vi "NMRvmefull3.vi"() -> ()   [LabVIEW 2013]
uses:
  <vilib>/Utility/file.llb/Read From Spreadsheet File (DBL).vi
  <vilib>/Analysis/NI_AALBase.lvlib
panel:
  in  "Real/quad Q curve":bool=TRUE
  out "Temperature":dbl(graph)=22.5
  out "+3V supply":dbl=3.026 format="%_4g"
  out "Temp (C)":dbl=22.5 format="%_4g"
  in  "RemovePed":bool=TRUE
  in  "IF / LOG Det":bool
  in  "Q curve file":string="realback213.txt"
  out "File name 2":string="C:\\users\\plm\\Desktop\\rssmt\\realback213.txt"
  in  "AutoBaseline":bool=TRUE
  out "RF OK":bool=TRUE
  out "Peak area (V-MHz)":sgl=0.008512556 format="%.5f"
  in  "Gauss Fit":bool=TRUE
  out "NMR Graph + Fit":cluster{cluster{dbl, "Numeric":dbl}[]}[](graph)=[{[{224.37, "Numeric"=-0.000659019047619289}, {224.372, "Numeric"=-0.001187546666660903}, {224.374, "Numeric"=-0.003239274285720313}, {224.376, "Numeric"=-0.004214201904762039}, {224.37800000000001, "Numeric"=-0.002912329523803976}, {224.38, "Numeric"=-0.007933657142862722}, {224.382, "Numeric"=-0.005878184761904778}, {224.38400000000001, "Numeric"=-0.00914591238094707}, {224.386, "Numeric"=-0.00463684000000517}, {224.388, "Numeric"=-0.0009509676190475541}, {224.39000000000001, "Numeric"=-0.004488295238090173}, {224.392, "Numeric"=-0.004948822857147612}, {224.394, "Numeric"=-0.0035325504761903404}, {224.39600000000002, "Numeric"=-0.0007394780952332926}, {224.398, "Numeric"=0.0009303942857099255}, {224.4, "Numeric"=0.004277066666666864}, {224.40200000000002, "Numeric"=0.0017005390476235753}, {224.404, "Numeric"=0.0039008114285674464}, {224.406, "Numeric"=0.003777883809524034}, {224.40800000000002, "Numeric"=0.004031756190480424}, {224.41, "Numeric"=0.0019624285714249347}, {224.412, "Numeric"=0.00796990095238121}, {224.41400000000002, "Numeric"=5.417333333726862e-05}, {224.416, "Numeric"=0.0012152457142824398}, {224.418, "Numeric"=-0.0023468819047616283}, {224.42000000000002, "Numeric"=-0.00023220952380592283}, {224.422, "Numeric"=0.003659262857139909}, {224.424, "Numeric"=0.0047275352380955005}, {224.426, "Numeric"=0.008272607619049287}, {224.428, "Numeric"=0.008894479999997358}, {224.43, "Numeric"=0.011693152380952624}, {224.432, "Numeric"=0.01246862476190608}, {224.434, "Numeric"=0.0106208971428548}, {224.436, "Numeric"=0.012149969523809723}, {224.438, "Numeric"=0.01675584190476286}, {224.44, "Numeric"=0.02263851428571223}, {224.442, "Numeric"=0.026497986666666827}, {224.444, "Numeric"=0.03243425904761961}, {224.446, "Numeric"=0.04374733142856964}, {224.448, "Numeric"=0.0529372038095239}, {224.45, "Numeric"=0.06540387619047636}, {224.452, "Numeric"=0.07984734857142704}, {224.454, "Numeric"=0.09986762095238097}, {224.456, "Numeric"=0.11866469333333307}, {224.458, "Numeric"=0.15183856571428445}, {224.46, "Numeric"=0.19398923809523802}, {224.462, "Numeric"=0.24311671047618982}, {224.464, "Numeric"=0.30252098285714174}, {224.466, "Numeric"=0.347502055238095}, {224.468, "Numeric"=0.3777599276190465}, {224.47, "Numeric"=0.3782945999999991}, {224.472, "Numeric"=0.35440607238095206}, {224.474, "Numeric"=0.29719434476190315}, {224.476, "Numeric"=0.24975941714285646}, {224.478, "Numeric"=0.19870128952380905}, {224.48, "Numeric"=0.16101996190475984}, {224.482, "Numeric"=0.13171543428571375}, {224.484, "Numeric"=0.10748770666666604}, {224.486, "Numeric"=0.08753677904761648}, {224.488, "Numeric"=0.0769626514285711}, {224.49, "Numeric"=0.06146532380952299}, {224.492, "Numeric"=0.05464479619047311}, {224.494, "Numeric"=0.04340106857142838}, {224.496, "Numeric"=0.041234140952379955}, {224.498, "Numeric"=0.034844013333334194}, {224.5, "Numeric"=0.02723068571428565}, {224.502, "Numeric"=0.02559415809523689}, {224.504, "Numeric"=0.015134430476191776}, {224.506, "Numeric"=0.017151502857142897}, {224.508, "Numeric"=0.013645375238093822}, {224.51, "Numeric"=0.008016047619049357}, {224.512, "Numeric"=0.015663520000000142}, {224.514, "Numeric"=0.01228779238095072}, {224.516, "Numeric"=0.005288864761906909}, {224.518, "Numeric"=0.010166737142857376}, {224.51999999999998, "Numeric"=0.007321409523806038}, {224.522, "Numeric"=0.008652881904764452}, {224.524, "Numeric"=0.003961154285714588}, {224.52599999999998, "Numeric"=0.004446226666662913}, {224.528, "Numeric"=0.002708099047621988}, {224.53, "Numeric"=-0.0015532285714282253}, {224.53199999999998, "Numeric"=0.0016622438095197614}, {224.534, "Numeric"=-0.00014548380952048717}, {224.536, "Numeric"=-0.002276411428571029}, {224.53799999999998, "Numeric"=6.946095237661282e-05}, {224.54, "Numeric"=0.00029213333333700424}, {224.542, "Numeric"=0.001291605714286121}, {224.54399999999998, "Numeric"=0.003967878095233438}, {224.546, "Numeric"=-0.0030790495238055193}, {224.548, "Numeric"=-0.0037491771428567293}, {224.54999999999998, "Numeric"=-0.0031425047619097436}, {224.552, "Numeric"=-0.005059032380948048}, {224.554, "Numeric"=-0.006498759999999599}, {224.55599999999998, "Numeric"=-0.0052616876190529505}, {224.558, "Numeric"=-0.005247815238090598}, {224.56, "Numeric"=-0.008557142857142475}, {224.56199999999998, "Numeric"=0.0013103295238038309}, {224.564, "Numeric"=-0.0059453980952331505}, {224.566, "Numeric"=-0.005024325714285373}, {224.56799999999998, "Numeric"=-0.006226453333339399}, {224.57, "Numeric"=-0.01565178095237573}]}, {[{224.37, "Numeric"=1.2216920919387119e-26}, {224.372, "Numeric"=1.2707531124356022e-25}, {224.374, "Numeric"=1.2602215540394123e-24}, {224.376, "Numeric"=1.1915682596026088e-23}, {224.37800000000001, "Numeric"=1.074180467048424e-22}, {224.38, "Numeric"=9.232554443628677e-22}, {224.382, "Numeric"=7.565764268347757e-21}, {224.38400000000001, "Numeric"=5.911123533707065e-20}, {224.386, "Numeric"=4.403252266347702e-19}, {224.388, "Numeric"=3.1272557579616753e-18}, {224.39000000000001, "Numeric"=2.1175785840334696e-17}, {224.392, "Numeric"=1.3671053194326456e-16}, {224.394, "Numeric"=8.414933959385655e-16}, {224.39600000000002, "Numeric"=4.9383941847663025e-15}, {224.398, "Numeric"=2.7631667539992904e-14}, {224.4, "Numeric"=1.474058566437982e-13}, {224.40200000000002, "Numeric"=7.497365525223633e-13}, {224.404, "Numeric"=3.635707470038474e-12}, {224.406, "Numeric"=1.6809526567726662e-11}, {224.40800000000002, "Numeric"=7.409831514948406e-11}, {224.41, "Numeric"=3.114207067787316e-10}, {224.412, "Numeric"=1.2478803346260637e-09}, {224.41400000000002, "Numeric"=4.7674340851587536e-09}, {224.416, "Numeric"=1.7365318588608352e-08}, {224.418, "Numeric"=6.030691537295004e-08}, {224.42000000000002, "Numeric"=1.99681475508499e-07}, {224.422, "Numeric"=6.303688449783224e-07}, {224.424, "Numeric"=1.897308734090218e-06}, {224.426, "Numeric"=5.4446199856763875e-06}, {224.428, "Numeric"=1.489647258961794e-05}, {224.43, "Numeric"=3.885846244500032e-05}, {224.432, "Numeric"=9.664381932133422e-05}, {224.434, "Numeric"=0.0002291653005566002}, {224.436, "Numeric"=0.000518095636666997}, {224.438, "Numeric"=0.001116753474559677}, {224.44, "Numeric"=0.0022950438712561385}, {224.442, "Numeric"=0.004496876629042055}, {224.444, "Numeric"=0.008400734433419424}, {224.446, "Numeric"=0.014962695593284949}, {224.448, "Numeric"=0.025409067505081276}, {224.45, "Numeric"=0.04113901748058781}, {224.452, "Numeric"=0.06350463222880787}, {224.454, "Numeric"=0.09346374892359874}, {224.456, "Numeric"=0.1311496966920382}, {224.458, "Numeric"=0.1754598225609385}, {224.46, "Numeric"=0.2238073695319673}, {224.462, "Numeric"=0.2721807344877579}, {224.464, "Numeric"=0.31559250621481655}, {224.466, "Numeric"=0.3488849894624623}, {224.468, "Numeric"=0.3677258738997204}, {224.47, "Numeric"=0.36953229107129204}, {224.472, "Numeric"=0.354051877915298}, {224.474, "Numeric"=0.3234206247194692}, {224.476, "Numeric"=0.28167922867646705}, {224.478, "Numeric"=0.23389893037116466}, {224.48, "Numeric"=0.18517738653314392}, {224.482, "Numeric"=0.13977643736304876}, {224.484, "Numeric"=0.10059265830727328}, {224.486, "Numeric"=0.06902158134856975}, {224.488, "Numeric"=0.04515333441124985}, {224.49, "Numeric"=0.028163138467571368}, {224.492, "Numeric"=0.016747831227365746}, {224.494, "Numeric"=0.009495599803450215}, {224.496, "Numeric"=0.005133014978954904}, {224.498, "Numeric"=0.0026455072873873718}, {224.5, "Numeric"=0.0012999651045567388}, {224.502, "Numeric"=0.0006090328646084895}, {224.504, "Numeric"=0.0002720420660815896}, {224.506, "Numeric"=0.00011585577912496795}, {224.508, "Numeric"=4.704198526856143e-05}, {224.51, "Numeric"=1.8211255302093487e-05}, {224.512, "Numeric"=6.721720126132654e-06}, {224.514, "Numeric"=2.3654145853830547e-06}, {224.516, "Numeric"=7.936342772979279e-07}, {224.518, "Numeric"=2.5387495830503464e-07}, {224.51999999999998, "Numeric"=7.742935028573666e-08}, {224.522, "Numeric"=2.251529631140118e-08}, {224.524, "Numeric"=6.2421761553258384e-09}, {224.52599999999998, "Numeric"=1.6499875819670289e-09}, {224.528, "Numeric"=4.1582599244703297e-10}, {224.53, "Numeric"=9.99145856172782e-11}, {224.53199999999998, "Numeric"=2.2889296881634745e-11}, {224.534, "Numeric"=4.999450980324916e-12}, {224.536, "Numeric"=1.0411144604004796e-12}, {224.53799999999998, "Numeric"=2.0670974178453588e-13}, {224.54, "Numeric"=3.9129987765540336e-14}, {224.542, "Numeric"=7.062277550488454e-15}, {224.54399999999998, "Numeric"=1.215251463338106e-15}, {224.546, "Numeric"=1.9937643473100612e-16}, {224.548, "Numeric"=3.1186583504921976e-17}, {224.54999999999998, "Numeric"=4.6510186053397055e-18}, {224.552, "Numeric"=6.613245651569734e-19}, {224.554, "Numeric"=8.965355910234511e-20}, {224.55599999999998, "Numeric"=1.1587952779623013e-20}, {224.558, "Numeric"=1.4280131290425803e-21}, {224.56, "Numeric"=1.6778146633486307e-22}, {224.56199999999998, "Numeric"=1.8794988861895673e-23}, {224.564, "Numeric"=2.0073655264081265e-24}, {224.566, "Numeric"=2.0440765317757311e-25}, {224.56799999999998, "Numeric"=1.984513896750819e-26}, {224.57, "Numeric"=1.8369504363521433e-27}]}]
  in  "Amp of Q curve":dbl=2.899999999999994 min=0.0 max=3.0 step=0.01 format="%_3f"
  in  "Subtract Q curve":bool=TRUE
  in  "Adjust Tune":bool
  out "Ped Offset":dbl(graph)=0.06850250000000084
  out "Pedestal Difference":dbl(graph)=-0.007803066666666664
  out "# Good Spectra":i32=29509
  in  "Quality cuts":bool=TRUE
  out "Pedestal OK":bool=TRUE
  out "Sweep #":i32=45
  out "1st Sweep":bool
  out "ADC volts OK":bool=TRUE
  out "Peak Height Distribution":cluster{"Y":dbl[], "Y":dbl[]}[](graph)=[{"Y"=[0.34871442808966735, 0.3488976491432983, 0.3490808701969293, 0.3492640912505603, 0.34944731230419124, 0.34963053335782224, 0.34981375441145324, 0.3499969754650842, 0.3501801965187152, 0.3503634175723462, 0.3505466386259771, 0.3507298596796081, 0.3509130807332391, 0.35109630178687007, 0.35127952284050107, 0.351462743894132, 0.351645964947763, 0.351829186001394, 0.35201240705502496, 0.35219562810865596, 0.35237884916228696, 0.3525620702159179, 0.3527452912695489, 0.3529285123231799, 0.35311173337681084, 0.35329495443044184, 0.3534781754840728, 0.3536613965377038, 0.3538446175913348, 0.35402783864496573, 0.35421105969859673, 0.35439428075222773, 0.3545775018058587, 0.3547607228594897, 0.3549439439131207, 0.3551271649667516, 0.3553103860203826, 0.3554936070740136, 0.35567682812764456, 0.35586004918127556, 0.3560432702349065, 0.3562264912885375, 0.3564097123421685, 0.35659293339579945, 0.35677615444943045, 0.35695937550306145, 0.3571425965566924, 0.3573258176103234, 0.3575090386639544, 0.35769225971758534, 0.35787548077121634, 0.3580587018248473, 0.3582419228784783, 0.3584251439321093, 0.3586083649857402, 0.3587915860393712, 0.3589748070930022, 0.35915802814663317, 0.35934124920026417, 0.35952447025389517, 0.3597076913075261, 0.3598909123611571, 0.3600741334147881, 0.36025735446841906, 0.36044057552205006, 0.360623796575681, 0.360807017629312, 0.360990238682943, 0.36117345973657394, 0.36135668079020494, 0.36153990184383594, 0.3617231228974669, 0.3619063439510979, 0.3620895650047289, 0.36227278605835983, 0.36245600711199083, 0.3626392281656218, 0.3628224492192528, 0.3630056702728838, 0.3631888913265147, 0.3633721123801457, 0.3635553334337767, 0.36373855448740766, 0.36392177554103866, 0.36410499659466966, 0.3642882176483006, 0.3644714387019316, 0.3646546597555626, 0.36483788080919355, 0.36502110186282455, 0.3652043229164555, 0.3653875439700865, 0.3655707650237175, 0.36575398607734844, 0.36593720713097944, 0.36612042818461044, 0.3663036492382414, 0.3664868702918724, 0.3666700913455034, 0.3668533123991343], "Y"=[24.0, 29.0, 32.0, 34.0, 34.0, 53.0, 50.0, 55.0, 70.0, 66.0, 63.0, 90.0, 88.0, 116.0, 110.0, 103.0, 137.0, 139.0, 177.0, 188.0, 191.0, 208.0, 220.0, 246.0, 251.0, 269.0, 294.0, 310.0, 304.0, 366.0, 401.0, 442.0, 412.0, 433.0, 437.0, 438.0, 496.0, 484.0, 531.0, 538.0, 550.0, 573.0, 590.0, 601.0, 617.0, 609.0, 585.0, 623.0, 652.0, 623.0, 610.0, 648.0, 648.0, 584.0, 616.0, 592.0, 652.0, 533.0, 589.0, 549.0, 539.0, 528.0, 504.0, 465.0, 524.0, 439.0, 441.0, 379.0, 358.0, 348.0, 329.0, 336.0, 272.0, 248.0, 270.0, 240.0, 216.0, 166.0, 192.0, 170.0, 175.0, 151.0, 123.0, 121.0, 113.0, 125.0, 102.0, 85.0, 77.0, 76.0, 66.0, 55.0, 58.0, 38.0, 47.0, 49.0, 31.0, 28.0, 28.0, 24.0]}]
  in  "# of Sweeps":i32=100000
  out "Std Dev (V)":dbl=0.0033690733987410434 format="%_2g"
  out "Peak mean (V)":dbl=0.35771809344101635 format="%_4g"
  out "Peak Height":dbl(graph)=0.3709256223473899
  in  "Raw Data":bool=TRUE
  in  "Tank RF":bool=TRUE
  in  "IF Atten (dB)":i8 min=0 max=31 step=1
  in  "IFoffset (V)":dbl=-1.3340288000000005 min=-5.0 max=5.0 step=0.001 format="%.4f"
  in  "Tune  (V)":dbl=1.091700000000001 min=0.0 max=5.0 step=0.001 format="%.4f"
  in  "Hi / Lo IF Gain":bool
  out "Voltage Array":sgl[](array[numeric])=[0.103, 0.1012, 0.0979, 0.0957, 0.0958, 0.0896, 0.0905, 0.0861, 0.0895, 0.0921, 0.0875, 0.086, 0.0864, 0.0882, 0.0889, 0.0913, 0.0878, 0.0891, 0.0881, 0.0875, 0.0846, 0.0898, 0.0811, 0.0815, 0.0772, 0.0786, 0.0818, 0.0822, 0.0851, 0.0851, 0.0873, 0.0875, 0.0851, 0.0861, 0.0902, 0.0956, 0.099, 0.1045, 0.1154, 0.1242, 0.1363, 0.1504, 0.1701, 0.1886, 0.2215, 0.2634, 0.3123, 0.3715, 0.4163, 0.4464, 0.4468, 0.4228, 0.3655, 0.318, 0.2669, 0.2292, 0.1999, 0.1757, 0.1558, 0.1453, 0.1299, 0.1232, 0.1121, 0.1101, 0.1039, 0.0965, 0.0951, 0.0849, 0.0872, 0.084, 0.0787, 0.0867, 0.0837, 0.0771, 0.0824, 0.08, 0.0818, 0.0776, 0.0786, 0.0774, 0.0737, 0.0775, 0.0763, 0.0748, 0.0778, 0.0787, 0.0804, 0.0838, 0.0775, 0.0776, 0.079, 0.0779, 0.0773, 0.0794, 0.0803, 0.0779, 0.0887, 0.0824, 0.0843, 0.0841, 0.0757] format="%.4f"
  in  "Invert Polarity":bool
  out "Pedestal Diff (V)":sgl=-0.0078030666 format="%.3f"
  out "Peak amp (V)":sgl=0.37092564 format="%.3f"
  in  "Save Data to File":bool
  in  "RF Level (dBm)":dbl=-1.0 min=-10.0 max=1.0 step=0.1 format="%.2f"
  out "SMT error out":errorcluster
  out "Sample RMS (V)":dbl=0.011017821782178215 format="%.4f"
  in  "# Sample/step":i32=200 min=1 max=1000 step=100
  in  "Step Width (MHz)":dbl=0.002 min=0.0 max=1000.0 step=0.0005 format="%.4f"
  in  "Freq Span (MHz)":dbl=0.2 min=0.0 max=3000.0 step=0.1 format="%.3f"
  in  "Center Freq (MHz)":dbl=224.47 min=0.005 max=6000.0 step=0.1 format="%.3f"
  in  "Sweep Mode":u16(ring)=3 items=["Off", "Single", "Auto", "Step"]
  in  "GPIB Addr (28)":refnum<visa-resource-name>="GPIB0::28::INSTR"
  # "E1039 Prototype NMR Control Panel"
  # "Settings"
  # "D\nA\nC"
  # "R\nF\n\nG\nE\nN \n\n+\n\nI\nF"
  # "A\nD\nC"
  # "D\nA\nT\nA\n\n+\n\nA \nN\nA\nL\nY\nS\nI\nS"
  # "I\n/\nO"
  # "Results"
  # "A\nv\ne\nr\na\ng\ne"
  # "S\nw\ne\ne\np"
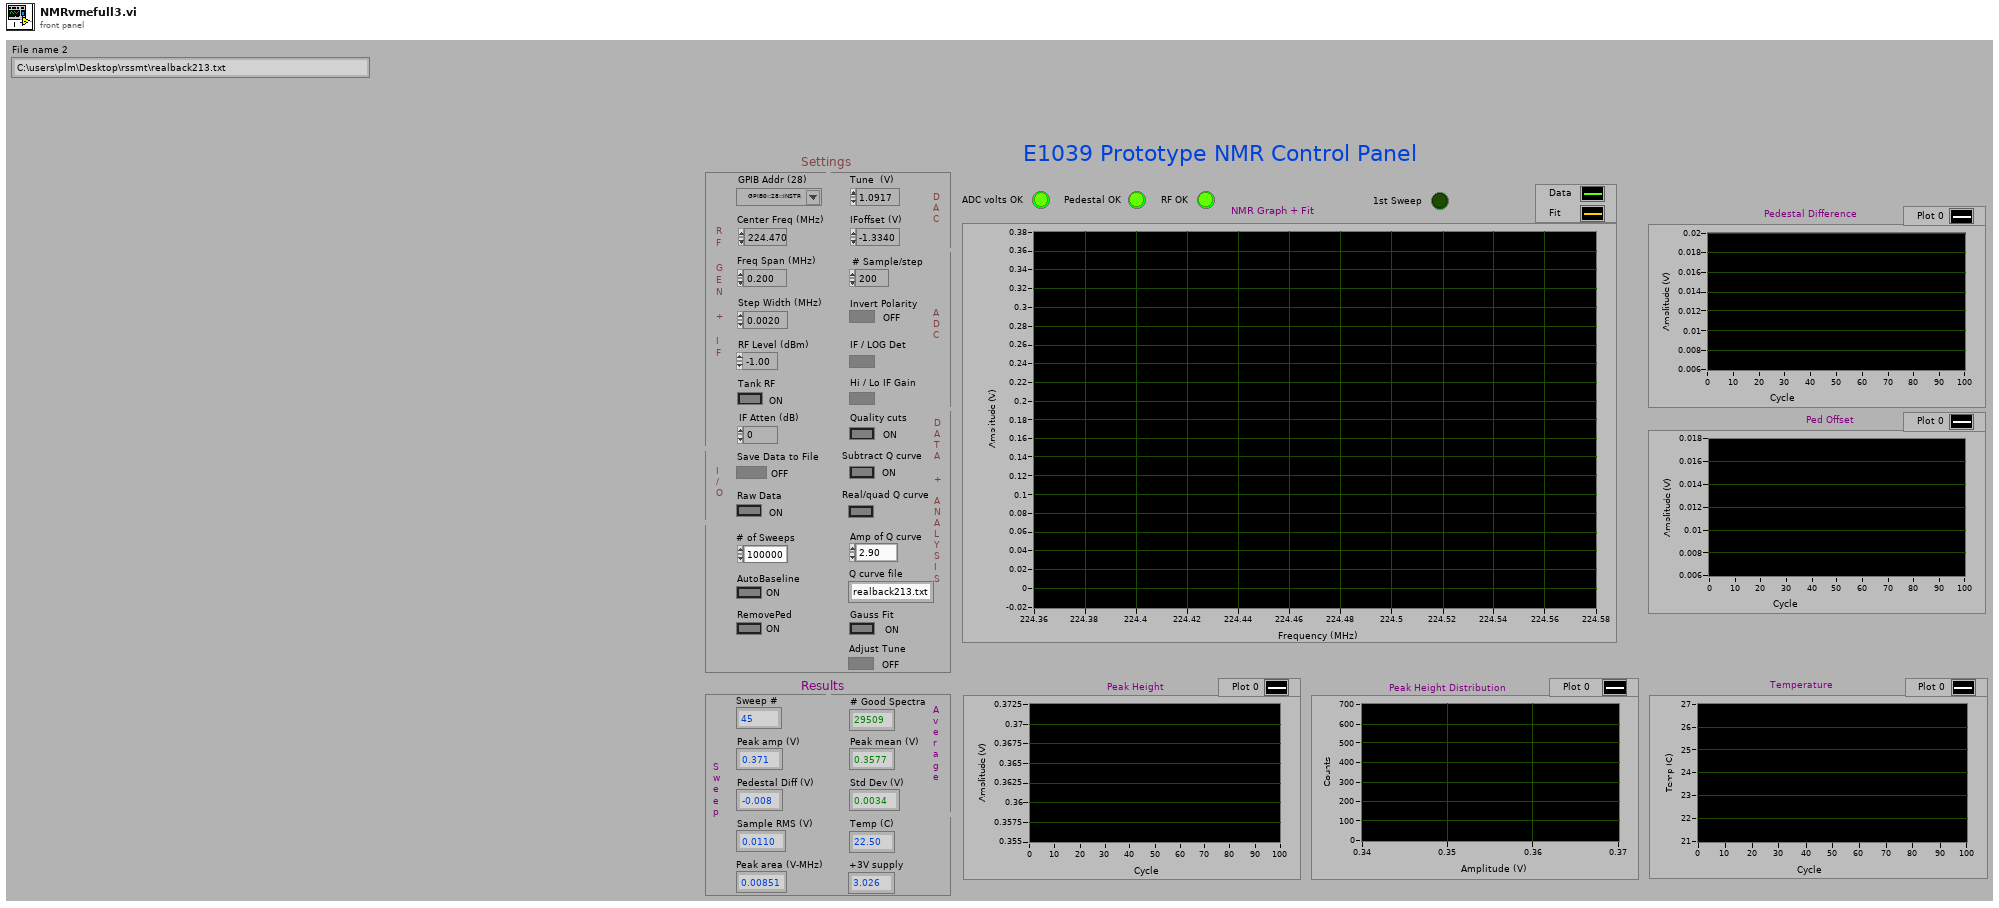
[diagram p1: front panel]
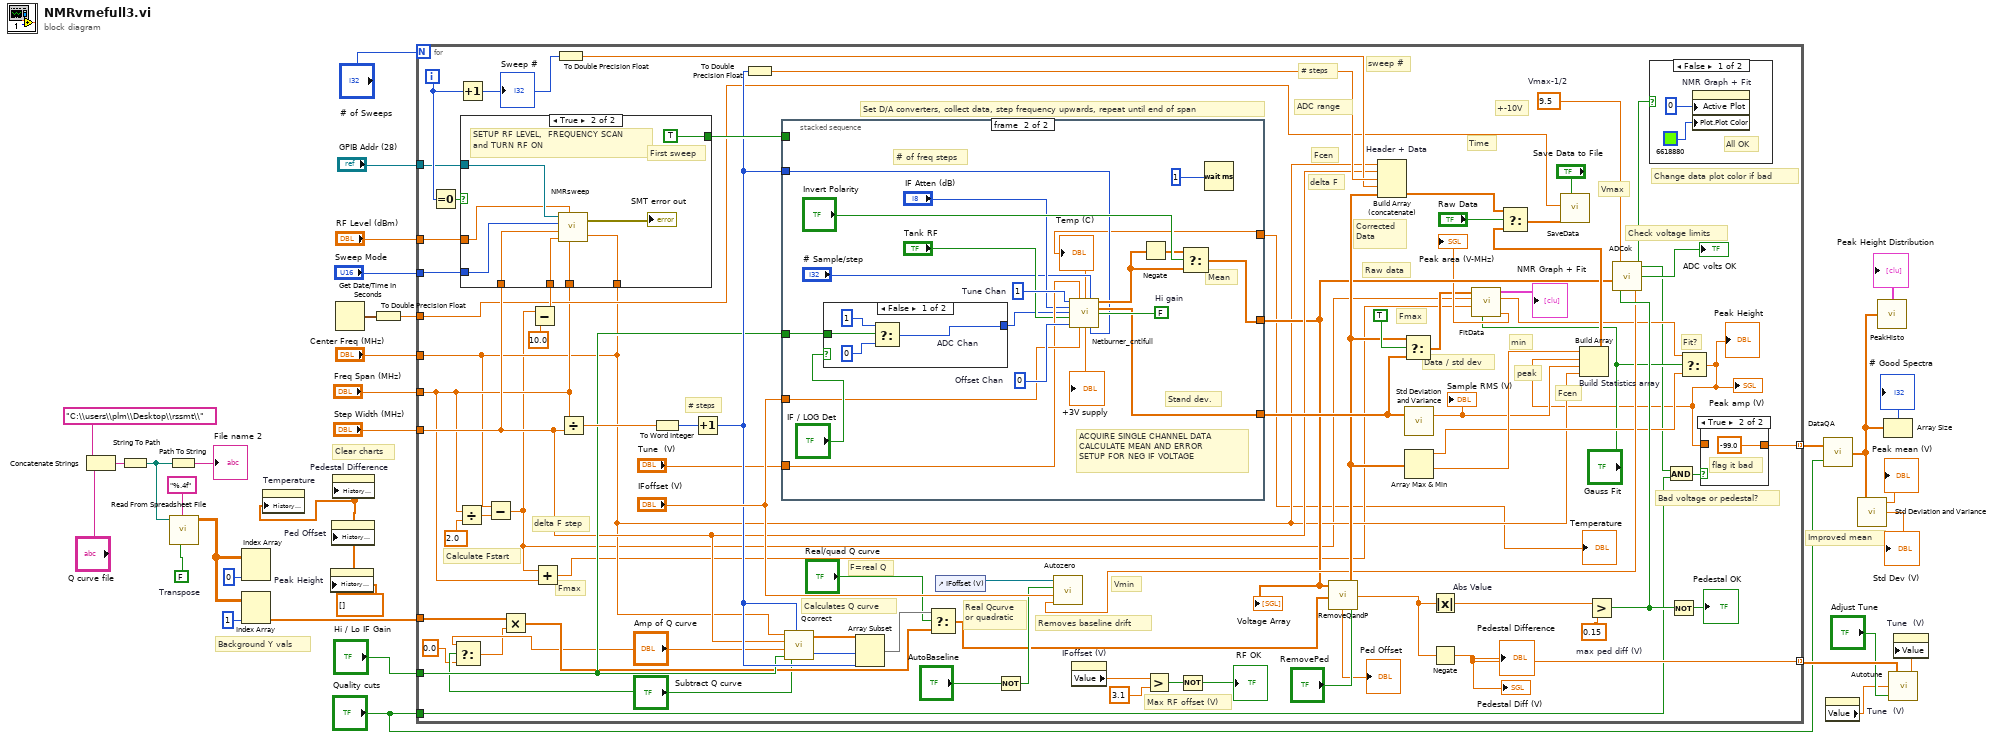
[diagram p0: block diagram]
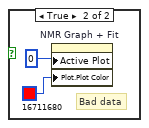
[diagram p2: hidden frame]
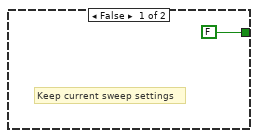
[diagram p4: hidden frame]
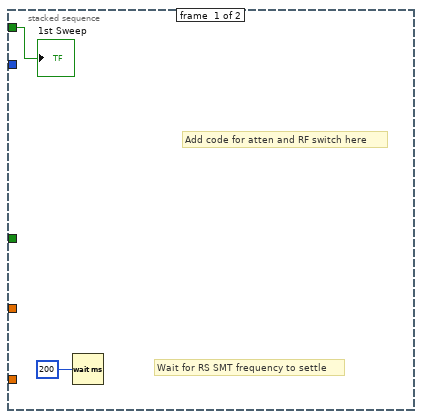
[diagram p5: hidden frame]
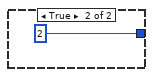
[diagram p6: hidden frame]
diagram:
  w9 = FALSE  # Transpose
  w1 = dbl[] []
  # "Background Y vals"
  # "Clear charts"
  # "Improved mean"
  n1 = Concatenate Strings "Concatenate Strings"("C:\\users\\plm\\Desktop\\rssmt\\", "Q curve file") -> (w12:string)
  n2 = String To Path(string=w12) -> (path=w8:path)
  n3 = Path To String(path=w8) -> (string=→"File name 2":string)
  n4 = call-poly <vilib>:"Read From Spreadsheet File.vi"("transpose (no:F)"=w9, "format (%.3f)"="%.4f", "file path (dialog if empty)"=w8) -> ("all rows"=w7:dbl[][])  [unwired: 4 in, 4 out]
  n5 = Index Array "Index Array"(array=w7, index (col)=0) -> ()  [unwired: 1 in, 1 out]
  n6 = Index Array(array=w7, index (col)=1) -> (element=w2:dbl[])  [unwired: 1 in]
  n7 = property on="Temperature" class="WFChart (strict)"("History Data"=w1) -> ()  [unwired: 2 in, 2 out]
  n8 = property on="Peak Height" class="WFChart (strict)"("History Data"=w1) -> ()  [unwired: 2 in, 2 out]
  n9 = property on="Ped Offset" class="WFChart (strict)"("History Data"=w1) -> ()  [unwired: 2 in, 2 out]
  n10 = property on="Pedestal Difference" class="WFChart (strict)"("History Data"=w1) -> ()  [unwired: 2 in, 2 out]
  n11 = Get Date/Time In Seconds() -> (seconds since 1Jan1904=w14:timestamp)
  n12 = To Double Precision Float(number=w14) -> (double precision float=w13:dbl)
  n13 = for {
    N: "# of Sweeps" -> [_]
    tunnel: [w94] -> w29 mode=indexing
    tunnel: "Quality cuts" -> [w71]
    tunnel: [w77] -> w26 mode=indexing
    tunnel: "Center Freq (MHz)" -> [w58]
    tunnel: "Freq Span (MHz)" -> [w64]
    tunnel: "Step Width (MHz)" -> [w70]
    tunnel: "Sweep Mode" -> [w81]
    tunnel: "Hi / Lo IF Gain" -> [w80]
    tunnel: "GPIB Addr (28)" -> [w79]
    tunnel: "RF Level (dBm)" -> [w78]
    tunnel: w13 -> [w65]
    tunnel: w2 -> [w43]
    i -> [w92]
    w75 = 9.5  # Vmax-1/2
    w95 = 0.15  # max ped diff (V)
    # "F=real Q"
    # "Real Qcurve\nor quadratic"
    # "+-10V"
    # "Vmax"
    # "Change data plot color if bad"
    # "Max RF offset (V)"
    # "Fmax"
    # "Fit?"
    # "Fmax"
    # "Time"
    # "Vmin"
    # "min"
    # "peak"
    # "Raw data"
    # "Corrected\nData"
    # "Fcen"
    # "delta F"
    # "# steps"
    # "ADC range"
    # "sweep #"
    # "Fcen"
    # "Set D/A converters, collect data, step frequency upwards, repeat until end of span"
    # "Calculates Q curve"
    # "Removes baseline drift"
    # "Bad voltage or pedestal?"
    # "Check voltage limits"
    # "Data / std dev"
    # "# steps"
    # "Calculate Fstart"
    # "delta F step"
    n14 = Equal To 0?(x=w92) -> (x = 0?=w97:bool)
    n15 = Select(t="Amp of Q curve", s="Subtract Q curve", f=0.0) -> (s? t:f=w38:dbl)
    n16 = Divide(x=w64, y=sgl 2.0) -> (x/y=w108:dbl)
    n17 = Increment(x=w92) -> (x+1=w82:i32)
    "Sweep #" <- w82
    n18 = Subtract(x=w58, y=w108) -> (x-y=w53:dbl)
    n19 = Multiply(x=w43, y=w38) -> (x*y=w42:dbl[])
    n20 = Subtract(x=w53, y=10.0) -> (x-y=w106:dbl)
    n21 = case shown="True" w97 {
      tunnel: w106 -> [_ w126]
      tunnel: w70 -> [_ w124]
      tunnel: w58 -> [_ w123]
      tunnel: w64 -> [_ w125]
      tunnel: [FALSE TRUE] -> w96
      tunnel: w81 -> [_ w120]
      tunnel: w79 -> [_ w119]
      tunnel: w78 -> [_ w118]
      frame False {
        # "Keep current sweep settings"
      }
      frame True {
        # "First sweep"
        # "SETUP RF LEVEL,  FREQUENCY SCAN\nand TURN RF ON"
        n22 = call "NMRsweep.vi"("Center Freq (MHz)"=w123, "Freq Span (MHz)"=w125, "RF Level (dBm)"=w118, "Foffset (MHz)"=w126, "Step Width (MHz)"=w124, "Sweep Mode"=w120, "GPIB Addr (28)"=w119) -> ("error out"=→"SMT error out":errorcluster)
      }
    }
    n23 = Add(x=w53, y=w64) -> (x+y=w52:dbl)
    n24 = To Double Precision Float(number=w82) -> (double precision float=w83:dbl)
    n25 = Divide(x=w64, y=w70) -> (x/y=w110:dbl)
    n26 = To Word Integer(number=w110) -> (16bit integer=w107:i16)
    n27 = Increment(x=w107) -> (x+1=w86:i16)
    n28 = To Double Precision Float(number=w86) -> (double precision float=w85:dbl)
    n29 = stacked-sequence {
      tunnel: [_ w134] -> w100
      tunnel: [_ w146] -> w68
      tunnel: w86 -> [_ w131]
      tunnel: "IFoffset (V)" -> [_ w141]
      tunnel: w80 -> [_ w144]
      tunnel: w96 -> [w127 _]
      tunnel: "Tune  (V)" -> [_ w139]
      tunnel: [_ w129] -> w34
      frame #0 {
        # "Add code for atten and RF switch here"
        # "Wait for RS SMT frequency to settle"
        n30 = Wait (ms)(milliseconds to wait=200) -> ()  [unwired: 1 out]
        "1st Sweep" <- w127
      }
      frame #1 {
        w136 = FALSE  # Hi gain
        w142 = 0  # Offset Chan
        w140 = 1  # Tune Chan
        # "Stand dev."
        # "Mean"
        # "ACQUIRE SINGLE CHANNEL DATA\nCALCULATE MEAN AND ERROR\nSETUP FOR NEG IF VOLTAGE"
        # "# of freq steps"
        n31 = case shown="False" "IF / LOG Det" {
          tunnel: w144 -> [w152 _]
          tunnel: [w149 2] -> w133
          frame False {
            n32 = Select "ADC Chan"(t=1, s=w152, f=0) -> (s? t:f=w149:i32)
          }
          frame True {
          }
        }
        n33 = call "Netburner_cntlfull.vi"("Tune DAC"=w140, "Tune Volt"=w139, "# Data"="# Sample/step", "IF Atten (dB)"="IF Atten (dB)", "NMR ADC"=w133, "Hi Gain"=w136, "Tank RF"="Tank RF", "Offset DAC"=w142, "Offset Volt"=w141, "# f steps"=w131) -> ("Temp (C)"=w129:dbl, "ADC value"=w135:dbl[], "ADC error"=w134:dbl[], "Volts"=→"+3V supply":dbl)  [unwired: 2 out]
        "Temp (C)" <- w129
        n34 = Negate(x=w135) -> (-x=w145:dbl[])
        n35 = Select(t=w145, s="Invert Polarity", f=w135) -> (s? t:f=w146:dbl[])
        n36 = Wait (ms)(milliseconds to wait=1) -> ()  [unwired: 1 out]
      }
    }
    "Voltage Array" <- w68
    "Temperature" <- w34
    n37 = call "Qcorrect.vi"("Subtract Q curve"="Subtract Q curve", "Nstep"=w86, "IF or Log"=w80, "Amp of Q curve"="Amp of Q curve", "Step Width (MHz)"=w70, "Center Freq (MHz)"=w58) -> ("Start"=w101:i32, "Array"=w102:dbl[])
    n38 = Array Subset "Array Subset"(array=w102, index=w101, length=w86) -> (w46:dbl[])
    n39 = Select(t=w46, s="Real/quad Q curve", f=w42) -> (s? t:f=w45:dbl[])
    n40 = control-ref of="IFoffset (V)"() -> (w74:refnum<vi>)
    n41 = Not(x="AutoBaseline") -> (.not. x?=w47:bool)
    n42 = property on="IFoffset (V)" class="DigNum (strict)"() -> ("Value"=w62:dbl)  [unwired: 2 in, 2 out]
    n43 = Greater?(x=w62, y=3.1) -> (0:w60:bool)
    n44 = Not(x=w60) -> (.not. x?=→"RF OK":bool)
    n45 = call "RemoveQandP.vi"("Subtract Ped?"="RemovePed", "Qcurve"=w45, "Raw data"=w68) -> ("Ped L-R"=w88:dbl, "Corrected data"=w84:dbl[], "Ped Offfset"=→"Ped Offset":dbl)
    n46 = Build Array (concatenate) "Header + Data"(w58, w70, w85, w83, w84) -> (w87:dbl[])
    n47 = Select(t=w84, s=TRUE, f=w100) -> (s? t:f=w54:dbl[])
    n48 = call <vilib>:"Std Deviation and Variance.vi"("X"=w100) -> ("mean"=w69:dbl)  [unwired: 1 in, 2 out]
    "Sample RMS (V)" <- w69
    n49 = Array Max & Min(array=w84) -> (max value=w63:dbl, min value=w99:dbl)  [unwired: 2 out]
    n50 = Absolute Value "Abs Value"(x=w88) -> (abs(x)=w90:dbl)
    n51 = Negate(x=w88) -> (-x=w77:dbl)
    "Pedestal Diff (V)" <- w77
    "Pedestal Difference" <- w77
    n52 = call "FitData.vi"("Fit?"="Gauss Fit", "Fmax"=w52, "Fmin"=w53, "Yarray"=w54) -> ("Peak Area (V-MHz)"=→"Peak area (V-MHz)":dbl, "Amplitude (V)"=w56:dbl, "NMR Graph + Fit"=→"NMR Graph + Fit":cluster{cluster{dbl, "Numeric":dbl}[]}[])  [unwired: 2 out]
    n53 = Greater?(x=w90, y=w95) -> (0:w76:bool)
    n54 = call "ADCok.vi"("PedOK"=w76, "Array"=w68, "Vmax-1/2"=w75) -> ("Vmin"=w73:dbl, "ADC voltages OK"=→"ADC volts OK":bool, "Allok"=w50:bool)
    n55 = call "Autozero.vi"("Vmin (V)"=w73, "IFoffset (V)"="IFoffset (V)", "IF or Log"=w47, "reference"=w74) -> ()
    n56 = case shown="False" w50 {
      frame False {
        # "All OK"
        n57 = property on="NMR Graph + Fit" class="XYGraph (strict)"("Active Plot"=0, "Plot.Plot Color"=u32 6618880) -> ()  [unwired: 2 in, 2 out]
      }
      frame True {
        # "Bad data"
        n58 = property on="NMR Graph + Fit" class="XYGraph (strict)"("Active Plot"=0, "Plot.Plot Color"=u32 16711680) -> ()  [unwired: 2 in, 2 out]
      }
    }
    n59 = And(x=w50, y=w71) -> (x .and. y?=w91:bool)
    n60 = Not(x=w76) -> (.not. x?=→"Pedestal OK":bool)
    n61 = Select(t=w56, s="Gauss Fit", f=w63) -> (s? t:f=w49:dbl)
    "Peak amp (V)" <- w49
    "Peak Height" <- w49
    n62 = Build Array "Build Statistics array"(w99, w49, w69, w58) -> (w105:dbl[])
    n63 = Select(t=w87, s="Raw Data", f=w105) -> (s? t:f=w66:dbl[])
    n64 = call "SaveData.vi"("Array"=w66, "Save Data to File"="Save Data to File", "Ext time (sec)"=w65) -> ()  [unwired: 1 out]
    n65 = case shown="True" w91 {
      tunnel: [w115 -99.0] -> w94
      tunnel: w49 -> [w115 _]
      frame False {
        # "Data OK"
      }
      frame True {
        # "flag it bad"
      }
    }
  }
  n66 = call "DataQA.vi"("Quality cuts"="Quality cuts", "Data In"=w29) -> ("Data Out"=w28:dbl[])
  n67 = property on="Tune  (V)" class="DigNum (strict)"() -> ("Value"=w17:dbl)  [unwired: 2 in, 2 out]
  n68 = call <vilib>:"Std Deviation and Variance.vi"("X"=w28) -> ("mean"=→"Peak mean (V)":dbl, "standard deviation"=→"Std Dev (V)":dbl)  [unwired: 1 in, 1 out]
  n69 = call "PeakHisto.vi"("Data Out"=w28) -> ("XY Graph"=→"Peak Height Distribution":cluster{"Y":dbl[], "Y":dbl[]}[])
  n70 = Array Size(array=w28) -> (size(s)=→"# Good Spectra":i32)
  n71 = call "Autotune.vi"("Adjust Tune"="Adjust Tune", "Tune Vin"=w17, "Pedestal Diff"=w26) -> ("Tune Vout"=w16:dbl)
  n72 = property on="Tune  (V)" class="DigNum (strict)"("Value"=w16) -> ()  [unwired: 2 in, 2 out]
